vi "Launcer.vi"() -> ()   [LabVIEW 2020]
uses:
  Processes/Counter/Counter.lvclass
  <vilib>/ActorFramework/Message Enqueuer/Message Enqueuer.lvclass/Message Enqueuer.ctl
  26a9e80c-2a9f-49e3-92ad-d9a001fec5f7.vi
  <vilib>/ActorFramework/Message Enqueuer/Enqueue.vi
  ServiceManager/ServiceManager/ServiceManager.lvclass
  C:/Program Files (x86)/National Instruments/LabVIEW 2020/vi.lib/ActorFramework/Actor/Actor.lvclass
  <vilib>/ActorFramework/Stop Msg/Stop Msg.lvclass
  C:/Program Files (x86)/National Instruments/LabVIEW 2020/vi.lib/ActorFramework/Message/Message.lvclass
  <vilib>/JDP Science/JSONtext/Variant to JSON Text.vi
  <vilib>/ActorFramework/Message Priority Queue/Priority Enqueue.vi
  <vilib>/ActorFramework/Actor/Actor.lvclass
panel:
  out "String":string
  in  "Count":u32
  in  "Send":bool
  in  "Connect":bool
  in  "stop":bool
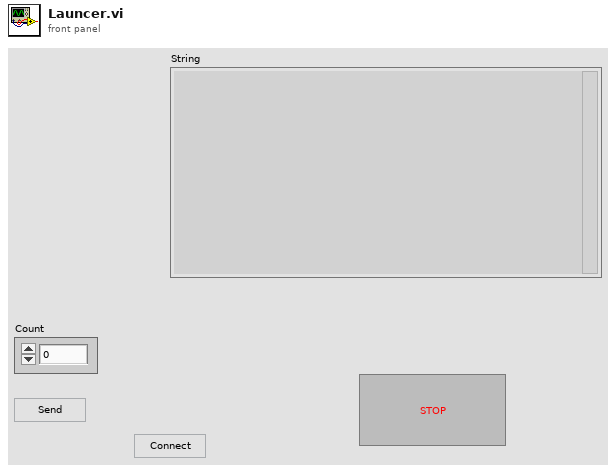
[diagram p1: front panel]
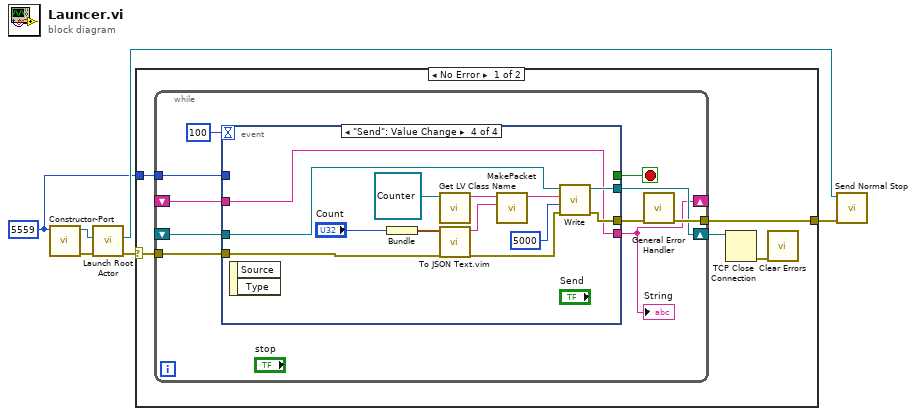
[diagram p0: block diagram]
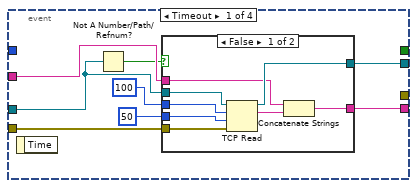
[diagram p2: hidden frame]
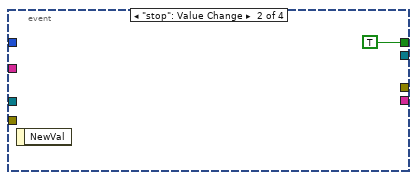
[diagram p4: hidden frame]
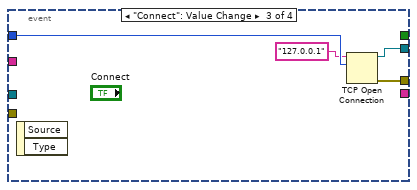
[diagram p5: hidden frame]
diagram:
  w1 = 5559 ("ListenerPort")
  n1 = call "Constructor-Port.vi"("ListenerPort"=w1) -> ("error out"=w5:errorcluster, "ServiceManager out"=w6:refnum<class "ServiceManager.lvclass">)  [unwired: 9 in]
  n2 = call <vilib>:"Launch Root Actor.vi"("error in (no error)"=w5, "Actor"=w6) -> ("error out"=w4:errorcluster, "Actor's Enqueuer"=w2:refnum<class "Message Enqueuer.lvclass">)  [unwired: 8 in]
  n3 = case shown="No Error" w4 {
    selector: w4 -> [w8 w57]
    tunnel: [w10 w57] -> w3
    tunnel: w1 -> [w11 _]
    frame No Error {
      n4 = while {
        tunnel: w11 -> [w20]
        tunnel: [w18] -> w10
        shift-right: [w17] -> w9
        shift-left: _ -> [w16]
        tunnel: w8 -> [w15]
        shift-right: [w13] -> _
        shift-left: _ -> [w12]
        stop <- w21 stop-if-true
        n5 = event shown="[3] \"Send\": Value Change" {
          selector: _ -> [_ _ _ _]
          dyn-events: _ -> [_ _ _ _]
          timeout: 100 -> [_ _ _ _]
          tunnel: [_ TRUE _ _] -> w21
          tunnel: w20 -> [_ _ w44 _]
          tunnel: [_ _ w42 w53] -> w19
          tunnel: [w26 _ w41 w54] -> w17
          tunnel: w16 -> [w23 _ _ w56]
          tunnel: w15 -> [w27 _ _ w55]
          tunnel: [w25 _ _ w45] -> w13
          tunnel: w12 -> [w24 _ _ w45]
          event Timeout {
            n6 = event-data() -> ()  [unwired: 1 in, 1 out]
            n7 = Not A Number/Path/Refnum?(number/path/refnum=w23) -> (NaN/Path/Refnum?=w22:bool)
            n8 = case shown="False" w22 {
              tunnel: 100 ("bytes to read") -> [w37 _]
              tunnel: 50 ("timeout ms (25000)") -> [w36 _]
              tunnel: w27 -> [w35 _]
              tunnel: [w34 w38] -> w26
              tunnel: [w32 w39] -> w25
              tunnel: w24 -> [w31 w39]
              tunnel: w23 -> [w30 w38]
              frame False {
                n9 = TCP Read(connection ID=w30, bytes to read=w37, error in (no error)=w35, 9:w36) -> (connection ID out=w34:refnum<k5>, data out=w33:string)  [unwired: 1 in, 1 out]
                n10 = Concatenate Strings(w31, w33) -> (w32:string)
              }
              frame True {
              }
            }
          }
          event "stop": Value Change {
            n11 = event-data() -> ()  [unwired: 1 in, 1 out]
          }
          event "Connect": Value Change {
            n12 = event-data() -> ()  [unwired: 1 in, 2 out]
            n13 = TCP Open Connection(address="127.0.0.1", remote port or service name=w44) -> (connection ID=w41:refnum<k5>, error out=w42:errorcluster)  [unwired: 3 in]
          }
          event "Send": Value Change {
            n14 = event-data() -> ()  [unwired: 1 in, 2 out]
            n15 = Bundle("Count"="Count") -> (w46:cluster{"Count":u32})  [unwired: 1 in]
            n16 = call <vilib>:"Get LV Class Name.vi"("object"=refnum<class "Counter.lvclass"> refnum ("TestProcesses.lvlib:Counter.lvclass")) -> ("class name"=w49:string)  [unwired: 9 in, 1 out]
            n17 = call "To JSON Text.vim"("Anything"=w46) -> ("<JSON>"=w48:string)  [unwired: 9 in, 1 out]
            n18 = call "MakePacket.vi"("Data"=w48, "STATE"=w49) -> ("<JSON>"=w51:string)  [unwired: 8 in, 1 out]
            n19 = call "Write.vi"("error in (no error)"=w55, "timeout ms (25000)"=5000, "data in"=w51, "connection ID"=w56) -> ("error out"=w53:errorcluster, "connection ID out"=w54:refnum<k5>)  [unwired: 6 in]
          }
        }
        "String" <- w13
        n20 = call <vilib>:"General Error Handler.vi"("error in (no error)"=w19) -> ("error out"=w18:errorcluster)  [unwired: 10 in, 4 out]
      }
      n21 = TCP Close Connection(connection ID=w9) -> (error out=w7:errorcluster)  [unwired: 2 in, 1 out]
      n22 = call <vilib>:"Clear Errors.vi"("error in (no error)"=w7) -> ()  [unwired: 5 in, 2 out]
    }
    frame Error {
    }
  }
  n23 = call <vilib>:"Send Normal Stop.vi"("error in (no error)"=w3, "Message Enqueuer"=w2) -> ()  [unwired: 9 in, 1 out]
